vi "Get LakeShore Configuration.vi"(8 "error in (no error)":errorcluster, 10 "Config in":T1={"Record Channels"=["A"], "Record raw signal"=FALSE, "Set point"=0.0, "Record heater"=FALSE, "Ramp rate"=0.0, "P"=1.0, "I"=0.0, "D"=60.0, "Control"=enum."Off", "P manual"=0.0, "Output #"=1}, 11 "VISA Resource Name":refnum<visa-resource-name>) -> (0 "error out":errorcluster, 2 "Config out":T1={"Record Channels"=["A"], "Record raw signal"=FALSE, "Set point"=0.0, "Record heater"=FALSE, "Ramp rate"=0.0, "P"=1.0, "I"=0.0, "D"=60.0, "Control"=enum."Off", "P manual"=0.0, "Output #"=0}, 3 "VISA Resource Name Out":refnum<visa-resource-name>)   [LabVIEW 2021]
uses:
  Temperature Controller Driver/T controller configuration.ctl
  Temperature Controller/Controls/Control Mode.ctl
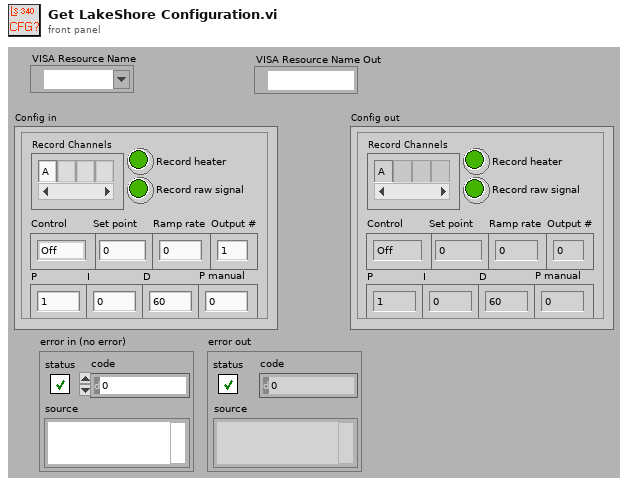
[diagram p1: front panel]
types:
  T1 = typedef "T controller configuration.ctl" = cluster{"Record Channels":string[], "Record raw signal":bool, "Set point":dbl, "Record heater":bool, "Ramp rate":dbl, "P":dbl, "I":dbl, "D":dbl, "Control":T2, "P manual":dbl, "Output #":i32}
  T2 = typedef "Control Mode.ctl" = enum16{"Off", "PID", "Ramp", "Manual", "Table"}
  T3 = typedef "LakeShore340 Mode.ctl" = enum16{"Off", "Manual PID", "Zone", "Open loop", "AutoTune PID", "AutoTune PI", "AutoTune P"}
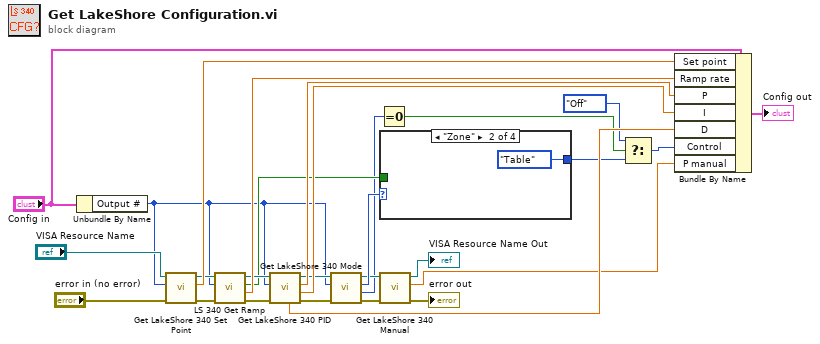
[diagram p0: block diagram]
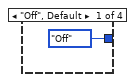
[diagram p2: hidden frame]
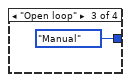
[diagram p3: hidden frame]
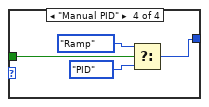
[diagram p4: hidden frame]
diagram:
  n1 = Unbundle By Name("Config in") -> ("Output #"=w6:i32)
  n2 = call "Get LakeShore 340 Set Point.vi"("error in (no error)"="error in (no error)", "Output #"=w6, "VISA Resource Name"="VISA Resource Name") -> ("error out"=w24:errorcluster, "Set point"=w26:dbl, "VISA Resource Name Out"=w25:refnum<visa-resource-name>)  [unwired: 6 in]
  n3 = call "LS 340 Get Ramp.vi"("error in (no error)"=w24, "Output #"=w6, "VISA resource name"=w25) -> ("error out"=w20:errorcluster, "Ramp rate, K/min"=w22:dbl, "Ramp on"=w13:bool, "VISA Resource Name Out"=w19:refnum<visa-resource-name>)  [unwired: 5 in]
  n4 = call "Get LakeShore 340 PID.vi"("error in (no error)"=w20, "Output #"=w6, "VISA Resource Name"=w19) -> ("error out"=w15:errorcluster, "I"=w17:dbl, "P"=w18:dbl, "VISA Resource Name Out"=w12:refnum<visa-resource-name>, "D"=w16:dbl)  [unwired: 4 in]
  n5 = call "Get LakeShore 340 Mode.vi"("error in (no error)"=w15, "Output #"=w6, "VISA Resource Name"=w12) -> ("error out"=w9:errorcluster, "on/off"=w5:i32, "Lake shore mode"=w14:T3, "VISA Resource Name Out"=w11:refnum<visa-resource-name>)  [unwired: 2 in, 3 out]
  n6 = Equal To 0?(x=w5) -> (x = 0?=w4:bool)
  n7 = case shown="\"Zone\"" w14 {
    tunnel: w13 -> [_ _ _ w35]
    tunnel: [Control_Mode."Off" ("Control") Control_Mode."Table" ("Control") Control_Mode."Manual" ("Control") w32] -> w3
    frame "Off", Default {
    }
    frame "Zone" {
    }
    frame "Open loop" {
    }
    frame "Manual PID" {
      n8 = Select(t=Control_Mode."Ramp" ("Control"), s=w35, f=Control_Mode."PID" ("Control")) -> (s? t:f=w32:T2)
    }
  }
  n9 = call "Get LakeShore 340 Manual.vi"("error in (no error)"=w9, "VISA Resource Name"=w11) -> ("error out"=→"error out":errorcluster, "Manual otput"=w10:dbl, "VISA Resource Name Out"=→"VISA Resource Name Out":refnum<visa-resource-name>)  [unwired: 7 in]
  n10 = Select(t=Control_Mode."Off", s=w4, f=w3) -> (s? t:f=w1:T2)
  n11 = Bundle By Name(cluster="Config in", "Set point"=w26, "Ramp rate"=w22, "P"=w18, "I"=w17, "D"=w16, "Control"=w1, "P manual"=w10) -> (→"Config out":T1)
